vi "HighlightTransferErrors.vi"(9 "File received":string, 11 "Sent/Recieved":refnum<vi>[](array[refnum])) -> (2 "diff":i16)   [LabVIEW 2024]
panel:
  out "Array 2":cluster{i32, i32}[](array[cluster])
  out "Array":cluster{i32, i32}[](array[cluster])
  out "Waveform Graph":i16[](graph)
  in  "File Sent":string
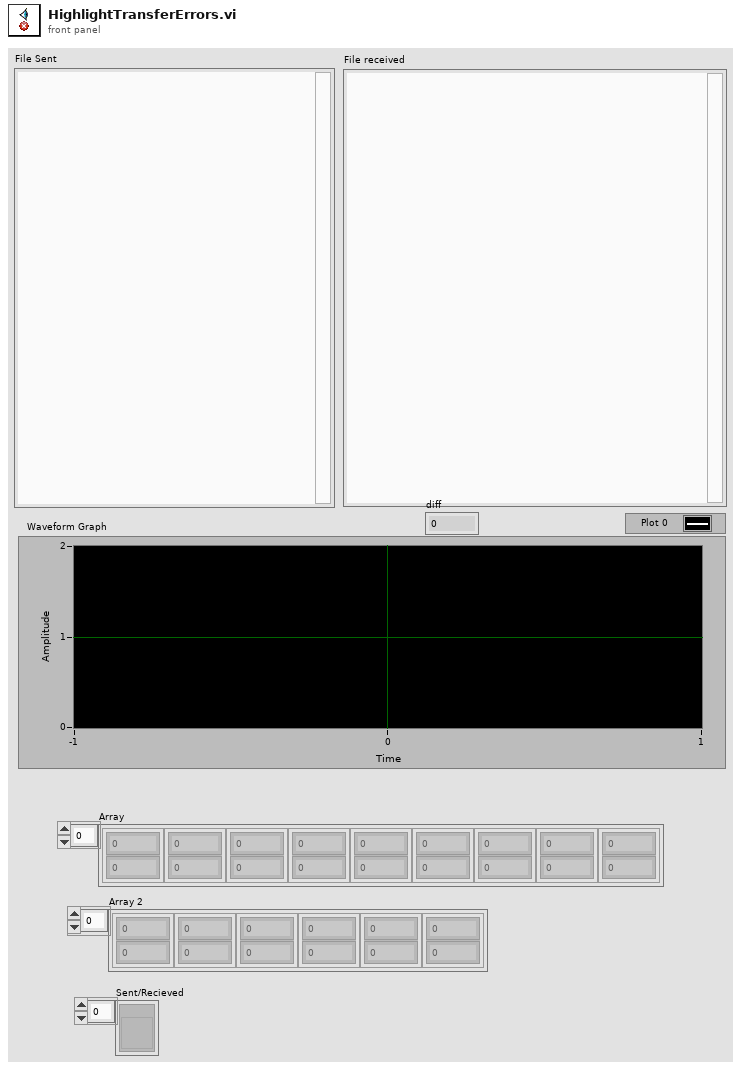
[diagram p1: front panel]
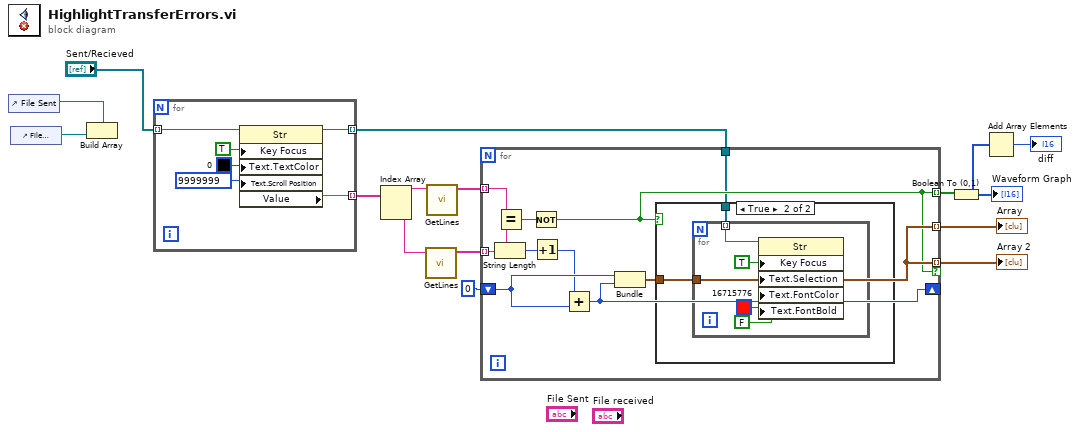
[diagram p0: block diagram]
diagram:
  n1 = control-ref of="File Sent"() -> (w8:refnum<vi>)
  n2 = control-ref of="File received"() -> (w7:refnum<vi>)
  n3 = Build Array(w8, w7) -> ()  [unwired: 1 out]
  n4 = for {
    tunnel: "Sent/Recieved" -> [w18] mode=indexing
    tunnel: [w17] -> w9 mode=indexing
    tunnel: [w16] -> w6 mode=indexing
    n5 = property on="Property Node" class="Str"(reference=w18, "Key Focus"=TRUE, "Text.TextColor"=u32 0 ("Text.Text Colors:Text Color"), "Text.Scroll Position"=u32 9999999) -> (reference out=w17:refnum<vi>, "Value"=w16:string)  [unwired: 1 in, 1 out]
  }
  n6 = Index Array(array=w6) -> (element #1=w5:string, element #2=w4:string)  [unwired: 2 in]
  n7 = call "GetLines.vi"("String"=w4) -> ("Array"=w14:string[])  [unwired: 10 in]
  n8 = call "GetLines.vi"("String"=w5) -> ("Array"=w15:string[])  [unwired: 10 in]
  n9 = for {
    tunnel: w15 -> [w31] mode=indexing
    tunnel: w14 -> [w30] mode=indexing
    shift-right: [w27] -> _
    shift-left: 0 -> [w28]
    tunnel: [w25] -> w12 mode=indexing if=w23
    tunnel: [w25] -> w11 mode=indexing
    tunnel: [w23] -> w10 mode=indexing
    tunnel: w9 -> [w22]
    n10 = String Length(string=w30) -> (length=w29:i32)
    n11 = Equal?(x=w31, y=w30) -> (x = y?=w24:bool)
    n12 = Not(x=w24) -> (.not. x?=w23:bool)
    n13 = Increment(x=w29) -> (x+1=w26:i32)
    n14 = Add(x=w26, y=w28) -> (x+y=w27:i32)
    n15 = Bundle(w28, w27) -> (w25:cluster{i32, i32})  [unwired: 1 in]
    n16 = case shown="True" w23 {
      tunnel: w25 -> [_ w33]
      tunnel: w22 -> [_ w32]
      frame False {
      }
      frame True {
        n17 = for {
          tunnel: w33 -> [w35]
          tunnel: w32 -> [w34] mode=indexing
          n18 = property on="Property Node" class="Str"(reference=w34, "Key Focus"=TRUE, "Text.Selection"=w35, "Text.FontColor"=u32 16715776 ("Text.Text Colors:Text Color"), "Text.FontBold"=FALSE ("Text.Font:Bold")) -> ()  [unwired: 1 in, 2 out]
        }
      }
    }
  }
  "Array" <- w11
  "Array 2" <- w12
  n19 = Boolean To (0,1)(Boolean=w10) -> (0, 1=w2:i16[])
  "Waveform Graph" <- w2
  n20 = Add Array Elements(numeric array=w2) -> (sum=→"diff":i16)
